vi "Connect.vi"(8 "error in (no error)":errorcluster, 10 "Channel(s)":string, 11 "Switch Instrument in":refnum<class "Switch Instrument.lvclass">) -> (0 "error out":errorcluster, 3 "Switch Instrument out":refnum<class "Switch Instrument.lvclass">)   [LabVIEW 2025, in "Switch.lvlib" / "Switch Instrument.lvclass"]
uses:
  Switch Instrument.lvclass
  Switch Instrument.lvclass/Switch Instrument.ctl
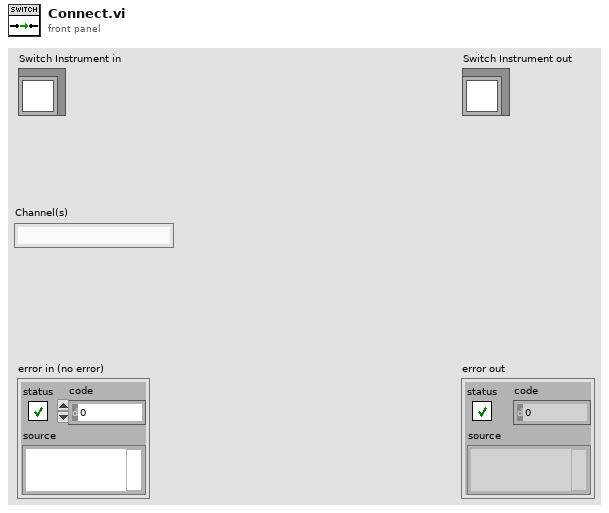
[diagram p1: front panel]
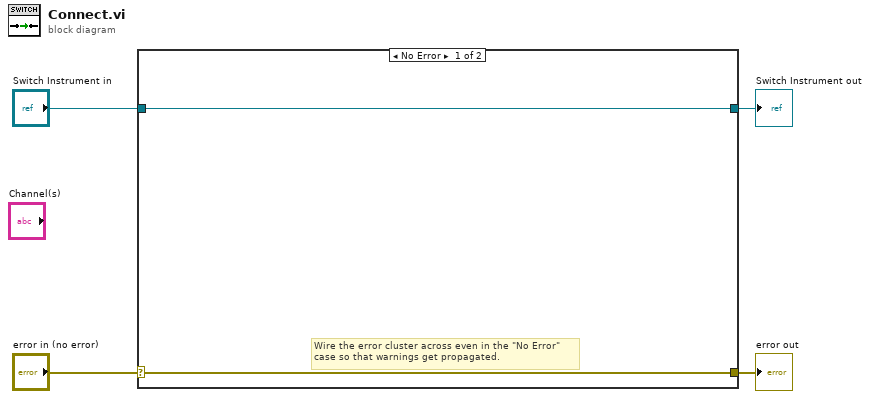
[diagram p0: block diagram]
diagram:
  n1 = case shown="No Error" "error in (no error)" {
    selector: "error in (no error)" -> [w5 w8]
    tunnel: [w5 w8] -> w3
    tunnel: [w6 w7] -> w1
    tunnel: "Switch Instrument in" -> [w6 w7]
    frame No Error {
      # "Wire the error cluster across even in the \"No Error\"\ncase so that warnings get propagated."
    }
    frame Error {
    }
  }
  "error out" <- w3
  "Switch Instrument out" <- w1
